vi "iniFilePathType.vi"(0 "refnum":T1, 1 "default value":path, 7 "section":string="RED", 11 "error in (no error)":errorcluster, 12 "key":string) -> (3 "Value":path, 4 "refnum out":T1, 6 "found?":bool, 8 "section dup":string="RED")   [LabVIEW 2015]
doc: "Same functionality than LabVIEW Native implementation but this version allows to interconnect same sections between, also default value, key and value in a cleaner way.\n\nAlso this implementation allows Python style comments on the configuration file, it parses out the #comments and left the key-value intact. Very convinient to comment out the .ini file\n\nDeveloped by Ezequiel Glz. plastilinapps.com"
uses:
  <vilib>/Utility/config.llb/Config Data RefNum.ctl
  <vilib>/Utility/config.llb/Read Key (Path).vi
  Python convention.vi
  <vilib>/Utility/config.llb/NI_LVConfig.lvlib
panel:
  out "error out":errorcluster
  # "Developed by Ezequiel Gonzalez\nPlastilinapps.com 2015"
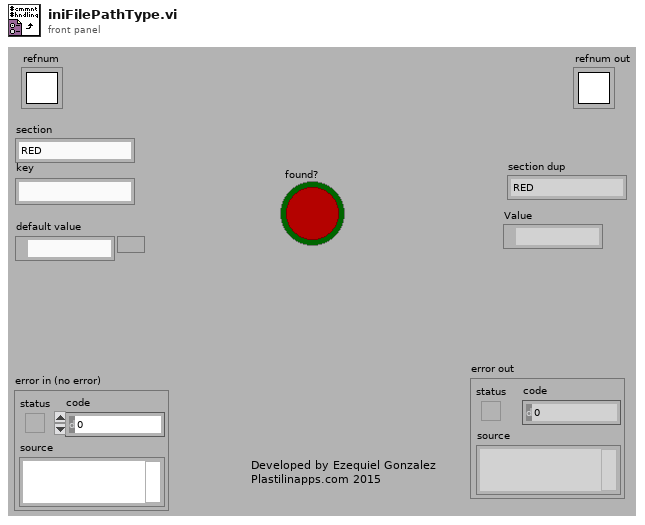
[diagram p1: front panel]
types:
  T1 = typedef "NI_LVConfig.lvlib/Config Data RefNum.ctl" = refnum<k1>
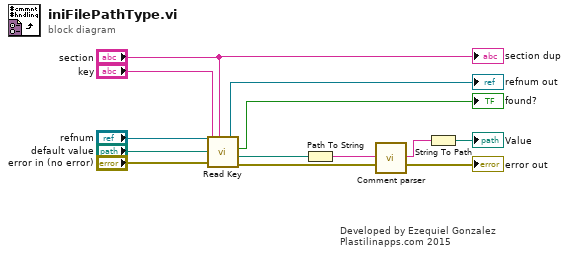
[diagram p0: block diagram]
diagram:
  # "Developed by Ezequiel Gonzalez\nPlastilinapps.com 2015"
  n1 = call-poly <vilib>:"Read Key.vi"("section"="section", "error in (no error)"="error in (no error)", "default value"="default value", "key"="key", "refnum"="refnum") -> ("error out"=w2:errorcluster, "value"=w6:path, "found?"=→"found?":bool, "refnum out"=→"refnum out":T1)  [unwired: 3 in]
  n2 = Path To String(path=w6) -> (string=w4:string)
  n3 = call-poly "Comment parser.vi"("String stream In"=w4, "error in"=w2) -> ("String parsed out"=w3:string, "error out"=→"error out":errorcluster)  [unwired: 24 in]
  n4 = String To Path(string=w3) -> (path=→"Value":path)
  "section dup" <- "section"
